vi "NormalizedFrequency.vi"() -> ()   [LabVIEW 2020]
uses:
  <vilib>/Analysis/NI_AALBase.lvlib
panel:
  in  "Waveform":T1(ring)
  out "Waveform Graph":dbl[](graph)
  in  "Frequency":dbl
  in  "Samples":dbl
  in  "Sampling Rate":dbl
  in  "F Type":enum16{"Cycle", "Sample"}(ring)
  # "digital frequency = analog frequency / sampling frequency"
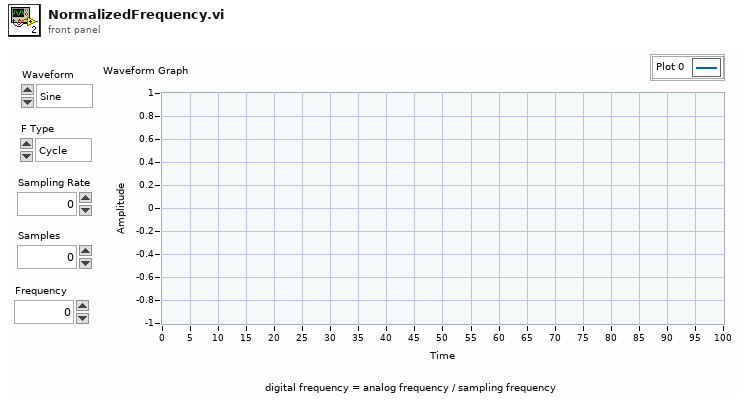
[diagram p1: front panel]
types:
  T1 = enum16{"Sine", "Square", "Sawtooth", "Triangle", "Arbitrary", "Chirp Pattern"}
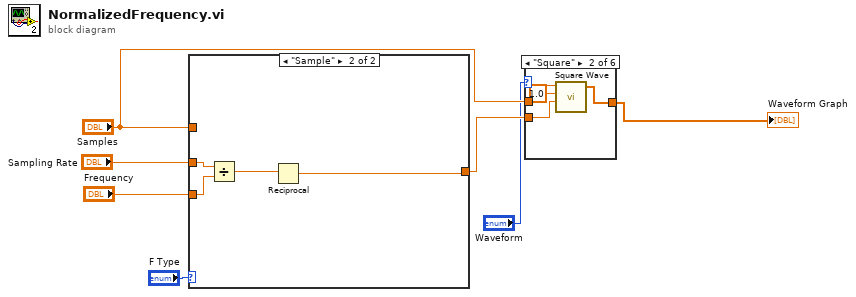
[diagram p0: block diagram]
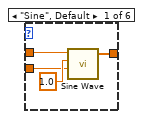
[diagram p2: hidden frame]
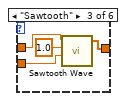
[diagram p3: hidden frame]
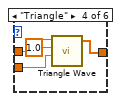
[diagram p4: hidden frame]
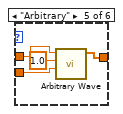
[diagram p5: hidden frame]
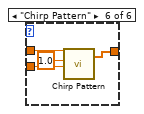
[diagram p6: hidden frame]
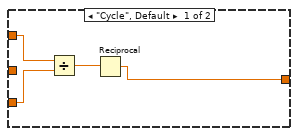
[diagram p7: hidden frame]
diagram:
  n1 = case shown="\"Sample\"" "F Type" {
    tunnel: "Sampling Rate" -> [_ w15]
    tunnel: "Frequency" -> [w10 w14]
    tunnel: "Samples" -> [w11 _]
    tunnel: [w8 w12] -> w3
    frame "Cycle", Default {
      n2 = Divide(x=w11, y=w10) -> (x/y=w9:dbl)
      n3 = Reciprocal(x=w9) -> (1/x=w8:dbl)
    }
    frame "Sample" {
      n4 = Divide(x=w15, y=w14) -> (x/y=w13:dbl)
      n5 = Reciprocal(x=w13) -> (1/x=w12:dbl)
    }
  }
  n6 = case shown="\"Square\"" "Waveform" {
    tunnel: "Samples" -> [w18 w22 w25 w29 w32 w38]
    tunnel: w3 -> [w17 w23 w26 w30 w34 w37]
    tunnel: [w16 w20 w27 w31 w35 w39] -> w2
    frame "Sine", Default {
      n7 = call <vilib>:"Sine Wave.vi"("samples"=w18, "amplitude"=1.0, "frequency"=w17) -> ("sine wave"=w16:dbl[])  [unwired: 2 in, 2 out]
    }
    frame "Square" {
      n8 = call <vilib>:"Square Wave.vi"("samples"=w22, "amplitude"=1.0, "frequency"=w23) -> ("square wave"=w20:dbl[])  [unwired: 3 in, 2 out]
    }
    frame "Sawtooth" {
      n9 = call <vilib>:"Sawtooth Wave.vi"("samples"=w25, "amplitude"=1.0, "frequency"=w26) -> ("sawtooth wave"=w27:dbl[])  [unwired: 2 in, 2 out]
    }
    frame "Triangle" {
      n10 = call <vilib>:"Triangle Wave.vi"("samples"=w29, "amplitude"=1.0, "frequency"=w30) -> ("triangle wave"=w31:dbl[])  [unwired: 2 in, 2 out]
    }
    frame "Arbitrary" {
      n11 = call <vilib>:"Arbitrary Wave.vi"("frequency"=w34, "amplitude"=1.0, "samples"=w32) -> ("arbitrary wave"=w35:dbl[])  [unwired: 4 in, 2 out]
    }
    frame "Chirp Pattern" {
      n12 = call <vilib>:"Chirp Pattern.vi"("f1"=w37, "amplitude"=1.0, "samples"=w38) -> ("Chirp Pattern"=w39:dbl[])  [unwired: 1 in, 1 out]
    }
  }
  "Waveform Graph" <- w2
